vi "CAN-CalpointMenu.vi"(8 "_ID":refnum<vi>, 9 "_Unit":refnum<vi>, 11 "_Name":refnum<vi>) -> ()   [LabVIEW 2016]
uses:
  <vilib>/addons/Software Calibration Management/xSCM/Controls/ID and Element.ctl
  <vilib>/addons/Software Calibration Management/xSCM/SCM-API.lvlib
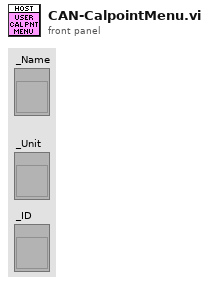
[diagram p1: front panel]
types:
  T1 = typedef "SCM-API.lvlib/ID and Element.ctl" = cluster{"ID":u32, "Element":i32[]}
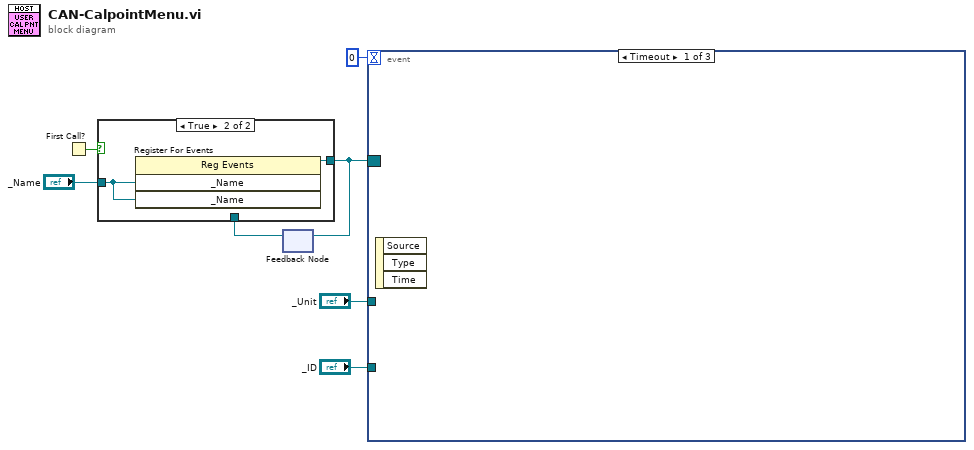
[diagram p0: block diagram]
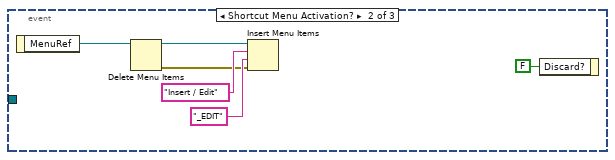
[diagram p2: hidden frame]
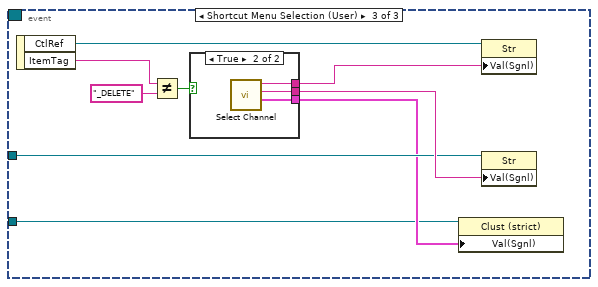
[diagram p3: hidden frame]
diagram:
  n1 = First Call?() -> (First Call?: T/F=w7:bool)
  n2 = feedback #1() -> (w5:refnum<event-registration>)  [unwired: 1 in]
  n3 = case shown="True" w7 {
    tunnel: "_Name" -> [_ w10]
    tunnel: [w8 w9] -> w6
    tunnel: w5 -> [w8 _]
    frame False {
    }
    frame True {
      n4 = register-events(w10, w10) -> (reference out=w9:refnum<event-registration>)  [unwired: 2 in, 1 out]
    }
  }
  n5 = feedback-in #1(w6) -> ()
  n6 = event shown="[0] Timeout" {
    selector: w6 -> [_ _ _]
    dyn-events: _ -> [_ _ _]
    timeout: 0 -> [_ _ _]
    tunnel: "_Unit" -> [_ _ w21]
    tunnel: "_ID" -> [_ _ w17]
    event Timeout {
      n7 = event-data() -> ()  [unwired: 1 in, 3 out]
    }
    event Shortcut Menu Activation? {
      n8 = event-data() -> ("MenuRef"=w12:refnum<k9>)  [unwired: 1 in]
      n9 = Delete Menu Items(9:w12) -> (0:w13:errorcluster, 3:w14:refnum<k9>)  [unwired: 3 in]
      n10 = Insert Menu Items(6:w13, 7:"_EDIT" ("format string"), 8:"Insert / Edit" ("item names"), 9:w14) -> ()  [unwired: 2 in, 3 out]
      n11 = event-data("Discard?"=FALSE) -> ()  [unwired: 1 in, 1 out]
    }
    event Shortcut Menu Selection (User) {
      n12 = event-data() -> ("CtlRef"=w19:refnum<vi>, "ItemTag"=w23:string)  [unwired: 1 in]
      n13 = Not Equal?(x=w23, y="_DELETE") -> (x != y?=w25:bool)
      n14 = case shown="True" w25 {
        tunnel: [_ w28] -> w20
        tunnel: [_ w27] -> w22
        tunnel: [_ w26] -> w18
        frame False {
        }
        frame True {
          n15 = call <vilib>:"Select Channel.vi"() -> ("ID"=w26:T1, "Units"=w27:string, "Name"=w28:string)  [unwired: 8 in, 1 out]
        }
      }
      n16 = property on="Property Node" class="Clust (strict)"(reference=w17, "Val(Sgnl)"=w18) -> ()  [unwired: 1 in, 2 out]
      n17 = property on="Property Node" class="Str"(reference=w19, "Val(Sgnl)"=w20) -> ()  [unwired: 1 in, 2 out]
      n18 = property on="Property Node" class="Str"(reference=w21, "Val(Sgnl)"=w22) -> ()  [unwired: 1 in, 2 out]
    }
  }
